vi "Single button PopUp Box.vi"(8 "Error In":errorcluster, 11 "Input Message":string="COMMUNICATION METHOD") -> (0 "Error Out":errorcluster, 3 "User DOne":bool)   [LabVIEW 2014]
uses:
  Buttons/Standard button.ctl
  Application Support/Stop Button/SubVI/Get Stop Button Status.vi
  Application Support/Front Panel/Window In Front/Bring Caller to Front.vi
panel:
  out "String":string="COMMUNICATION METHOD"
  in  "Done":T1
  in  "Join Mission":bool
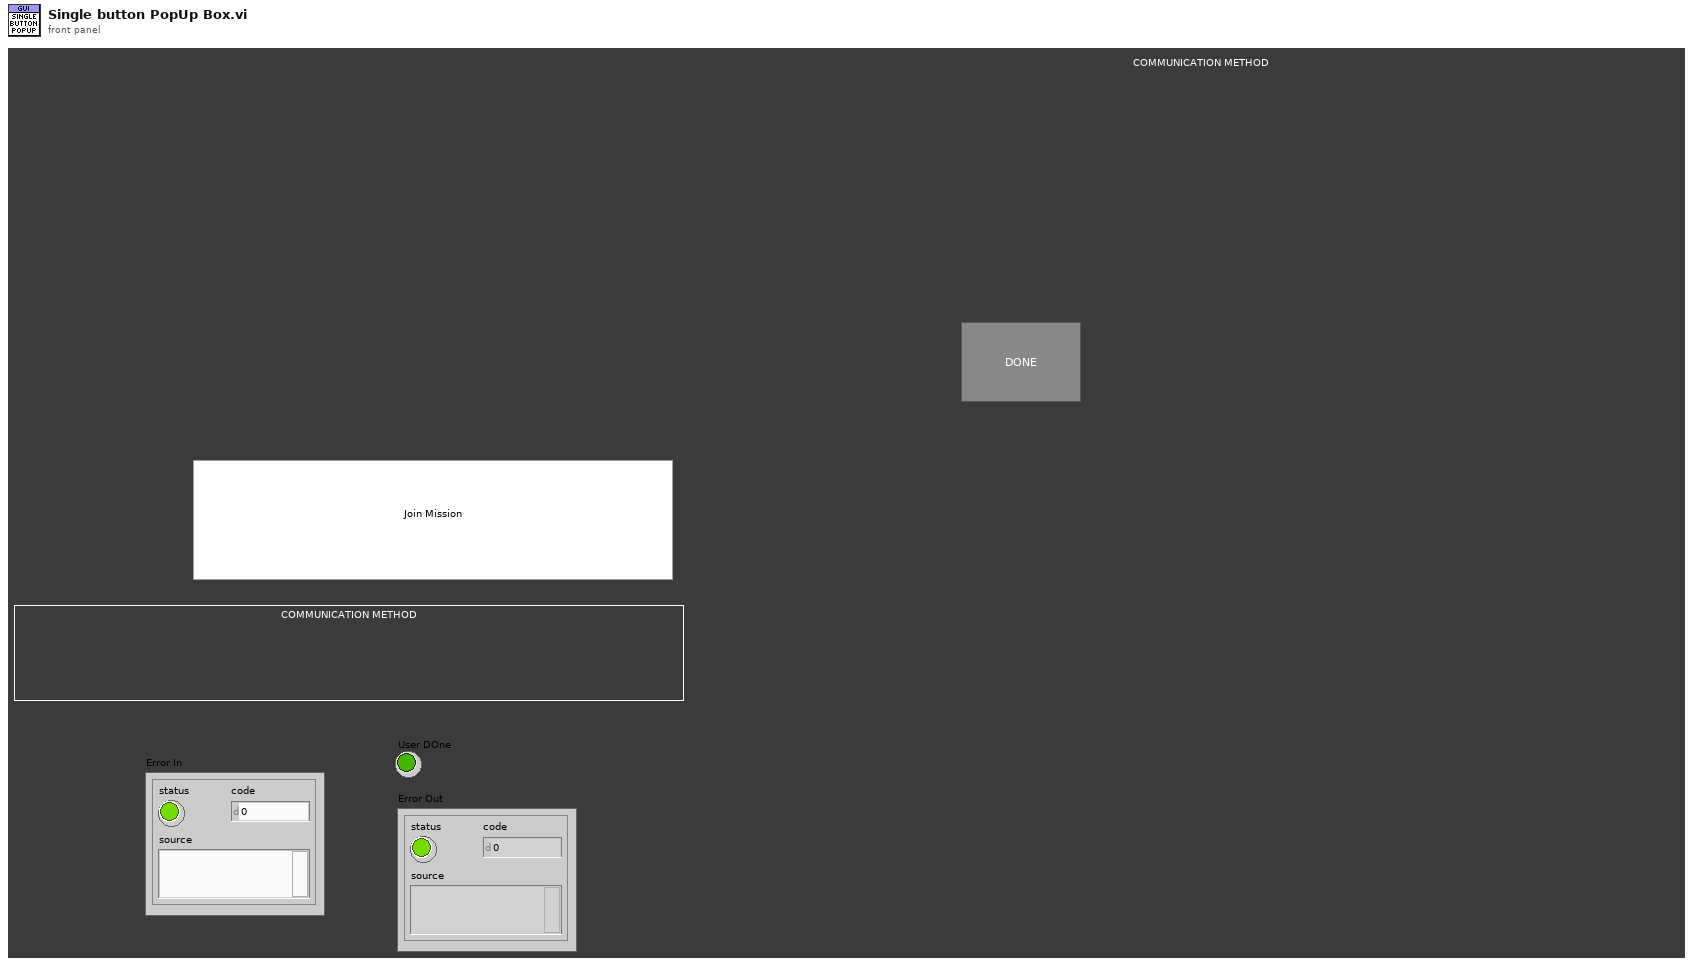
[diagram p1: front panel]
types:
  T1 = typedef "Standard button.ctl" = bool
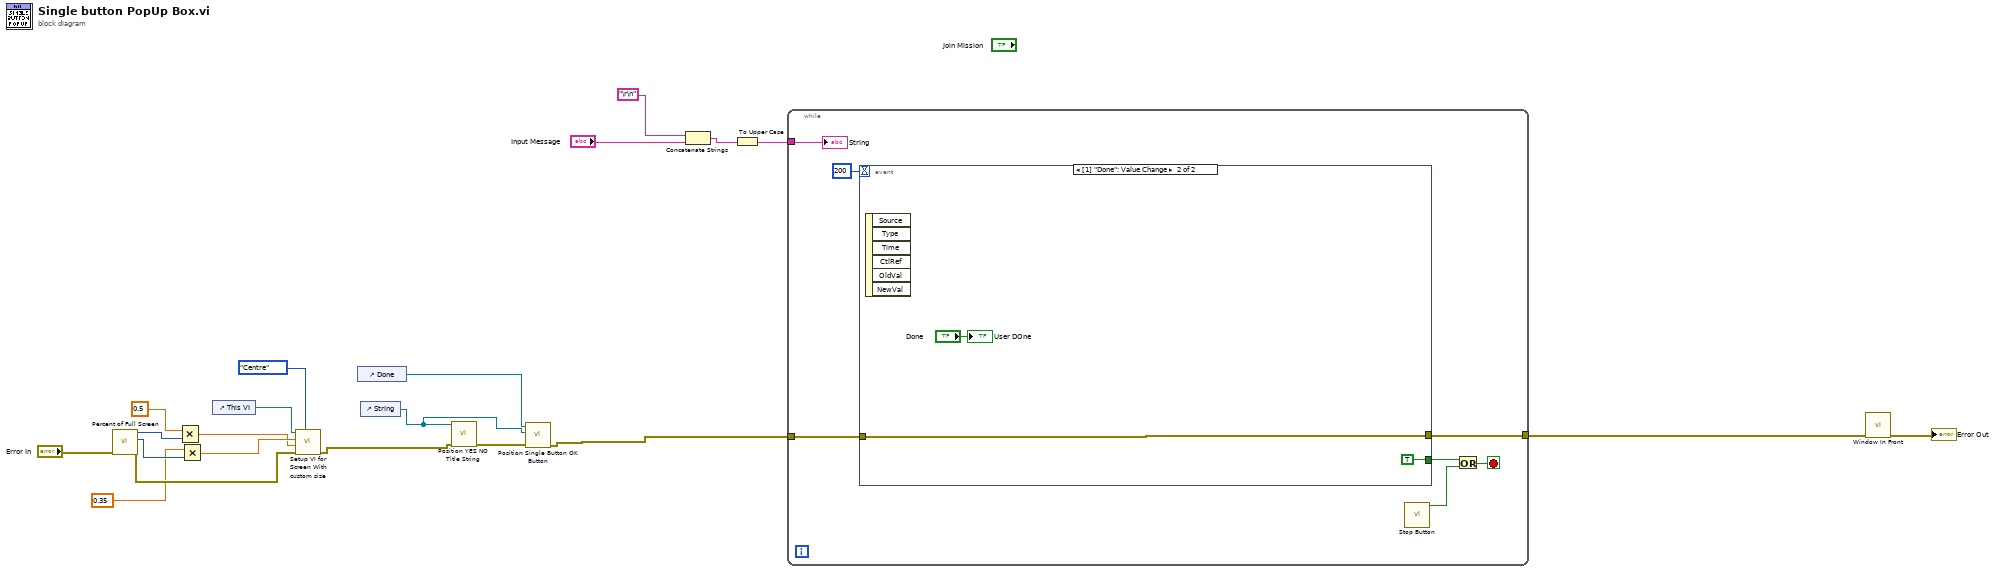
[diagram p0: block diagram]
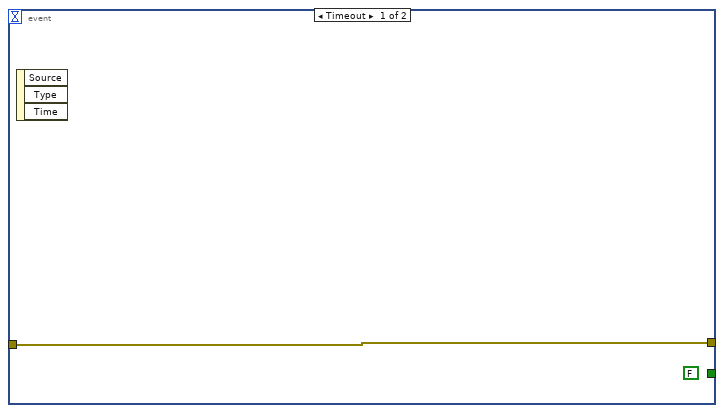
[diagram p2: hidden frame]
diagram:
  n1 = call "Percent of Full Screen.vi"("error in (no error)"="Error In") -> ("error out"=w11:errorcluster, "Bottom"=w15:i16, "Right"=w16:i16)  [unwired: 8 in]
  n2 = Multiply(x=0.5, y=w16) -> (x*y=w12:dbl)
  n3 = Multiply(x=0.35, y=w15) -> (x*y=w13:dbl)
  n4 = control-ref of="This VI"() -> (w18:refnum<vi>)
  n5 = call "Setup VI for Screen With custom size.vi"("Position"=enum16{"Top Left", "Centre"}."Centre", "Error In"=w11, "Width"=w12, "Height"=w13, "This VI"=w18) -> ("Error Out"=w10:errorcluster)  [unwired: 5 in, 1 out]
  n6 = control-ref of="Done"() -> (w3:refnum<vi>)
  n7 = control-ref of="String"() -> (w4:refnum<vi>)
  n8 = call "Position YES NO Title String.vi"("error in (no error)"=w10, "String Ref"=w4) -> ("error out"=w5:errorcluster)  [unwired: 9 in]
  n9 = call "Position Single Button OK Button.vi"("error in (no error)"=w5, "Message"=w4, "Button Ref"=w3) -> ("error out"=w6:errorcluster)  [unwired: 8 in]
  n10 = Concatenate Strings("\r\n", "Input Message") -> (w2:string)
  n11 = To Upper Case(1:w2) -> (0:w1:string)
  n12 = while {
    tunnel: w6 -> [w25]
    tunnel: [w24] -> w20
    tunnel: w1 -> [w22]
    stop <- w27 stop-if-true
    n13 = event shown="[1] \"Done\": Value Change" {
      selector: _ -> [_ _]
      dyn-events: _ -> [_ _]
      timeout: 200 -> [_ _]
      tunnel: [_ TRUE ("x")] -> w26
      tunnel: w25 -> [w29 w32]
      tunnel: [w29 w32] -> w24
      event Timeout {
        (unwired) FALSE ("x")
        n14 = event-data() -> ()  [unwired: 1 in, 3 out]
      }
      event Value Change {
        n15 = event-data() -> ()  [unwired: 1 in, 6 out]
        "User DOne" <- "Done"
      }
    }
    n16 = call-poly "Stop Button.vi"() -> ("Stop ButtonOut"=w28:bool)  [unwired: 10 in, 1 out]
    n17 = Or(x=w26, y=w28) -> (x .or. y?=w27:bool)
    "String" <- w22
  }
  n18 = call-poly "Window In Front.vi"("Error In"=w20) -> ("Error Out"=→"Error Out":errorcluster)  [unwired: 10 in]
